vi "FRCts20_WebMethods_Events_POST.vi"(7 "httpRequestID":u32) -> ()   [LabVIEW 2014, in "FRCts20_WebMethods.lvlib"]
doc: "<B>POST</B> a new competition resource\n\n<B>Required Data : </B>\n<Competition>\n <Name><B>string</B></Name>\n <Start_Date><B>YYYY-MM-DD</B></Start_Date>\n <Duration><B>uInt</B></Duration>\n</Competition>\n\nhttp://<server address>:<port>/FRCts/competition/\n\n{requires authentication}"
uses:
  FRCts20_WebMethods.lvlib
  <vilib>/wsapi/NI_WebServices.lvlib
  Backend/source/VI Source/FRCts20_Backend_API/FRCts20_Backend_API_Event.vi
  FRCts20_WebMethods_ReadData_Events.vi
  Backend/source/VI Source/FRCts20_Backend_API/FRCts20_Backend_API_Command_Event.ctl
  FRCts20_WebMethods_Redirect_Competition.vi
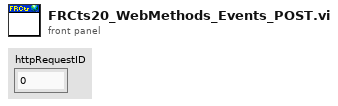
[diagram p1: front panel]
types:
  T1 = typedef "FRCts20_WebMethods.lvlib/FRCts20_WebMethods_ctl_singleEvent.ctl" = cluster{"Team":T2[], "Issue Count":i32, "Location":string, "Start Date ":timestamp}
  T2 = typedef "FRCts20_WebMethods.lvlib/FRCts20_WebMethods_ctl_teamIdentifier.ctl" = cluster{"Team Nickname":string, "Team Number ":u32, "UniqueId":u32}
  T3 = typedef "FRCts20_Backend_API.lvlib/FRCts20_Backend_API_Command_Event.ctl" = string
  T4 = typedef "FRCts20_Backend_API.lvlib/FRCts20_Backend_API_Event.ctl" = cluster{"Event Index":u32, "Name":string, "Start Time":timestamp, "End Time":timestamp, "Teams":cluster{"Team Index":u32, "Team Number":u32, "Requests":cluster{"Request Number":u32, "Description":string}[], "Has Open Issue":bool}[], "SWType":T5, "APIReturn":string}
  T5 = typedef "FRCts20_Backend_API.lvlib/FRCts20_Backend_API_SW.ctl" = string
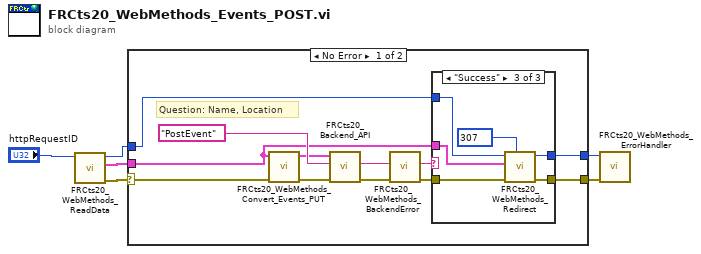
[diagram p0: block diagram]
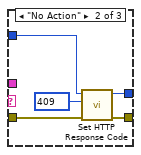
[diagram p3: hidden frame]
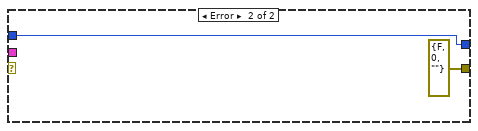
[diagram p4: hidden frame]
diagram:
  n1 = call-poly "FRCts20_WebMethods_ReadData.vi"("httpRequestID"="httpRequestID") -> ("error out"=w6:errorcluster, "Single Event out"=w1:T1, "httpRequestID out"=w2:u32)  [unwired: 8 in]
  n2 = case shown="No Error" w6 {
    selector: w6 -> [w10 _]
    tunnel: w1 -> [w7 _]
    tunnel: w2 -> [w16 w33]
    tunnel: [w15 errorcluster {"status"=FALSE, "code"=0, "source"=""} ("error out")] -> w5
    tunnel: [w14 w33] -> w4
    frame No Error {
      # "Question: Name, Location"
      n3 = call "FRCts20_WebMethods_Convert_Events_PUT.vi"("error in (no error)"=w10, "Single Event in"=w7) -> ("error out"=w9:errorcluster, "Event In"=w8:T4)  [unwired: 8 in]
      n4 = call-poly "FRCts20_Backend_API.vi"("error in (no error)"=w9, "Command"=T3 "PostEvent", "Event In"=w8) -> ("error out"=w13:errorcluster, "Status"=w12:string)  [unwired: 6 in, 1 out]
      n5 = call "FRCts20_WebMethods_BackendError.vi"("error in (no error)"=w13, "Status"=w12) -> ("error out"=w17:errorcluster, "Status out"=w18:string)  [unwired: 8 in]
      n6 = case shown="\"Success\"" w18 {
        tunnel: w17 -> [w19 w22 w31]
        tunnel: w16 -> [w20 w23 w30]
        tunnel: [w19 w25 w28] -> w15
        tunnel: [w20 w24 w27] -> w14
        tunnel: w7 -> [_ _ w26]
        frame "Backend Error", Default {
          # "`"
        }
        frame "No Action" {
          w21 = 409 items=["100"=100, "101"=101, "200"=200, "201"=201, "202"=202, "203"=203, "204"=204, "205"=205, "206"=206, "300"=300, "301"=301, "302"=302, "303"=303, "304"=304, "305"=305, "306"=306, "307"=307, "400"=400, "401"=401, "402"=402, "403"=403, "404"=404, "405"=405, "406"=406, "407"=407, "408"=408, "409"=409, "410"=410, "411"=411, "412"=412, "413"=413, "414"=414, "415"=415, "416"=416, "417"=417, "500"=500, "501"=501, "502"=502, "503"=503, "504"=504, "505"=505] ("response code (200)")
          n7 = call <vilib>:"Set HTTP Response Code.vi"("error in (no error)"=w22, "response code (200)"=w21, "httpRequestID"=w23) -> ("error out"=w25:errorcluster, "httpRequestID out"=w24:u32)  [unwired: 7 in]
        }
        frame "Success" {
          w29 = 307 items=["100"=100, "101"=101, "200"=200, "201"=201, "202"=202, "203"=203, "204"=204, "205"=205, "206"=206, "300"=300, "301"=301, "302"=302, "303"=303, "304"=304, "305"=305, "306"=306, "307"=307, "400"=400, "401"=401, "402"=402, "403"=403, "404"=404, "405"=405, "406"=406, "407"=407, "408"=408, "409"=409, "410"=410, "411"=411, "412"=412, "413"=413, "414"=414, "415"=415, "416"=416, "417"=417, "500"=500, "501"=501, "502"=502, "503"=503, "504"=504, "505"=505] ("response code (200)")
          n8 = call-poly "FRCts20_WebMethods_Redirect.vi"("response code (200)"=w29, "error in (no error)"=w31, "Single Event"=w26, "httpRequestID"=w30) -> ("error out"=w28:errorcluster, "httpRequestID out"=w27:u32)  [unwired: 6 in]
        }
      }
    }
    frame Error {
    }
  }
  n9 = call "FRCts20_WebMethods_ErrorHandler.vi"("error in"=w5, "LabVIEW Web Service Request"=w4) -> ()  [unwired: 8 in, 2 out]
